vi "Set ICAN.vi"(10 "ICAN":refnum<class "ICAN.lvclass">, 11 "CANopen in":refnum<class "CANopen.lvclass">) -> (3 "CANopen out":refnum<class "CANopen.lvclass">)   [LabVIEW 2024, in "canopen.lvlib" / "CANopen.lvclass"]
uses:
  CANopen.lvclass
  HAL/HAL/Protocols/ICAN/ICAN.lvclass
  CANopen.lvclass/CANopen.ctl
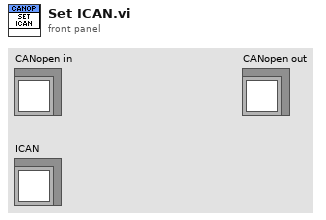
[diagram p1: front panel]
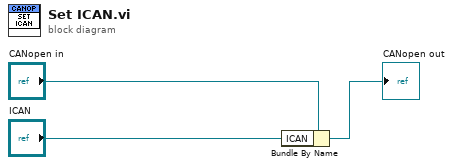
[diagram p0: block diagram]
diagram:
  n1 = Bundle By Name(cluster="CANopen in", "ICAN"="ICAN") -> (→"CANopen out":refnum<class "CANopen.lvclass">)
